vi "Voronoi_Range.vi"(9 "Centers":dbl[][](array[numeric]), 10 "Y":dbl[](array[numeric]), 11 "X":dbl[](array[numeric])) -> (3 "Range":dbl[](array[numeric]))   [LabVIEW 2020, in "NI_AAL_Geometry.lvlib"]
uses:
  <vilib>/Analysis/NI_AAL_Geometry.lvlib
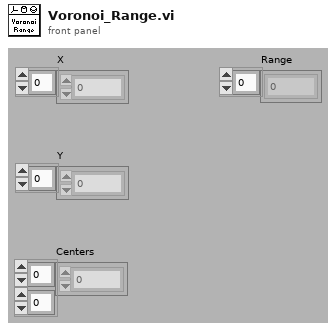
[diagram p1: front panel]
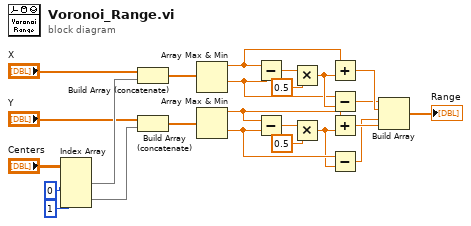
[diagram p0: block diagram]
diagram:
  n1 = Index Array(array="Centers", index (col) #1=0 ("disabled index (col)"), index (col) #2=1 ("index (col)")) -> (element #1=w5:dbl[], element #2=w3:dbl[])  [unwired: 2 in]
  n2 = Build Array (concatenate)("X", w5) -> (w2:dbl[])
  n3 = Build Array (concatenate)("Y", w3) -> (w1:dbl[])
  n4 = Array Max & Min(array=w2) -> (max value=w13:dbl, min value=w14:dbl)  [unwired: 2 out]
  n5 = Array Max & Min(array=w1) -> (max value=w18:dbl, min value=w17:dbl)  [unwired: 2 out]
  n6 = Subtract(x=w13, y=w14) -> (x-y=w11:dbl)
  n7 = Subtract(x=w18, y=w17) -> (x-y=w20:dbl)
  n8 = Multiply(x=w11, y=0.5) -> (x*y=w15:dbl)
  n9 = Multiply(x=w20, y=0.5) -> (x*y=w16:dbl)
  n10 = Add(x=w13, y=w15) -> (x+y=w22:dbl)
  n11 = Subtract(x=w14, y=w15) -> (x-y=w21:dbl)
  n12 = Add(x=w18, y=w16) -> (x+y=w24:dbl)
  n13 = Subtract(x=w17, y=w16) -> (x-y=w23:dbl)
  n14 = Build Array(w21, w22, w23, w24) -> (→"Range":dbl[])
